vi "Connection Status Monitor.vi"(6 "Module ID":i32=-1, 8 "error in":errorcluster, 10 "Acquisition Polling Time (ms* in":i32, 11 "VISA Refnum in":refnum<visa-resource-name>) -> (0 "error out":errorcluster, 2 "Acquisition Polling Time (ms* out":i32, 3 "VISA Refnum out":refnum<visa-resource-name>)   [LabVIEW 2020, in "RaspberryPiPico.lvlib"]
uses:
  RaspberryPiPico.lvlib
  a7f0f2bc-83fd-499f-a02e-86742517cef5.vi
  <instrlib>/HandsOnPi2040/HandsOnPi2040.lvlib
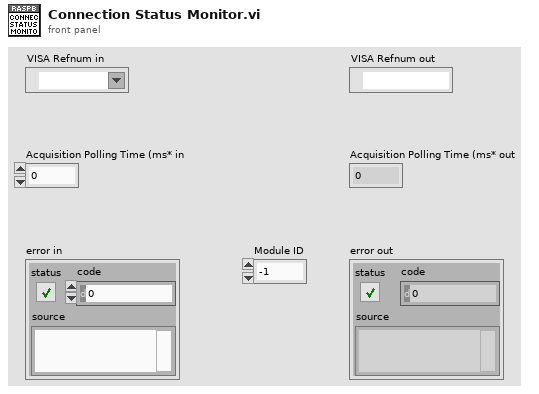
[diagram p1: front panel]
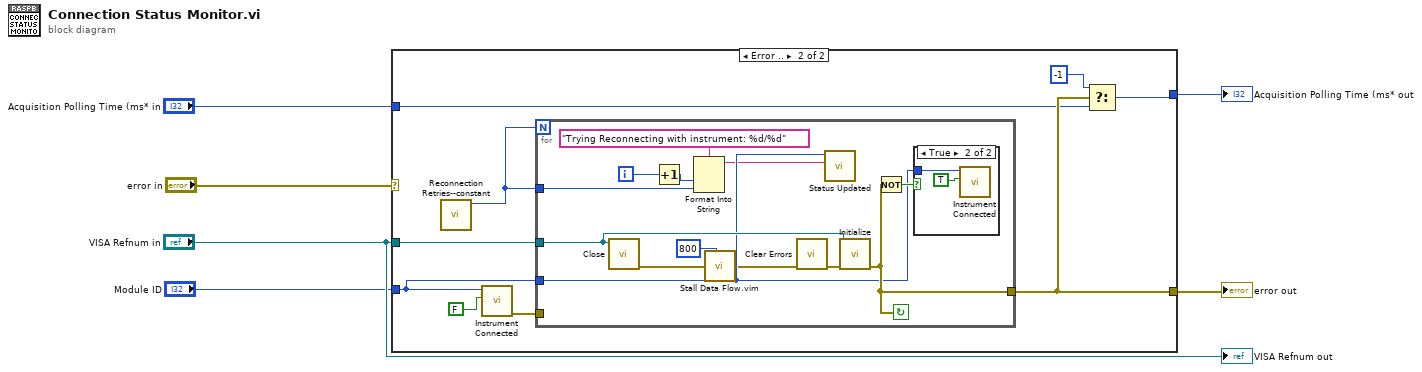
[diagram p0: block diagram]
diagram:
  n1 = case shown="Error .." "error in" {
    selector: "error in" -> [w8 _]
    tunnel: [w7 w15] -> w4
    tunnel: "Acquisition Polling Time (ms* in" -> [w7 w14]
    tunnel: "VISA Refnum in" -> [_ w12]
    tunnel: "Module ID" -> [_ w10]
    tunnel: [w8 w16] -> w5
    frame No Error {
    }
    frame Error {
      n2 = call "Reconnection Retries--constant.vi"() -> ("Number of Retries"=w9:i32)  [unwired: 11 in]
      n3 = call "Instrument Connected.vi"("Instrument Connection Status"=FALSE, "Module ID"=w10) -> ("error out"=w17:errorcluster)  [unwired: 9 in]
      n4 = for {
        N: w9 -> [_]
        tunnel: w12 -> [w27]
        tunnel: w17 -> [_]
        tunnel: w10 -> [w25]
        tunnel: [w28] -> w16
        tunnel: w9 -> [w22]
        i -> [w24]
        stop <- w28 continue-if-true
        n5 = call <instrlib>:"Close.vi"("VISA resource name"=w27) -> ("error out"=w30:errorcluster)  [unwired: 10 in]
        n6 = Increment(x=w24) -> (x+1=w18:i32)
        n7 = Format Into String(format string="Trying Reconnecting with instrument: %d/%d", w18, w22) -> (resulting string=w23:string)  [unwired: 2 in, 1 out]
        n8 = call "Stall Data Flow.vim"("value in"=w30, "milliseconds to wait"=u32 800) -> ("value out"=w20:errorcluster)  [unwired: 1 out]
        n9 = call <vilib>:"Clear Errors.vi"("error in (no error)"=w20) -> ("error out"=w29:errorcluster)  [unwired: 5 in, 1 out]
        n10 = call "Status Updated.vi"("Status"=w23, "Module ID"=w25) -> ()  [unwired: 9 in, 1 out]
        n11 = call <instrlib>:"Initialize.vi"("error in (no error)"=w29, "VISA resource name"=w27) -> ("error out"=w28:errorcluster)  [unwired: 7 in, 2 out]
        n12 = Not(x=w28) -> (.not. x?=w26:bool)
        n13 = case shown="True" w26 {
          tunnel: w25 -> [_ w32]
          frame False {
          }
          frame True {
            n14 = call "Instrument Connected.vi"("Instrument Connection Status"=TRUE, "Module ID"=w32) -> ()  [unwired: 9 in, 1 out]
          }
        }
      }
      n15 = Select(t=-1, s=w16, f=w14) -> (s? t:f=w15:i32)
    }
  }
  "Acquisition Polling Time (ms* out" <- w4
  "error out" <- w5
  "VISA Refnum out" <- "VISA Refnum in"
